vi "Loan_Calculator.vi"() -> ()   [LabVIEW 2022 SP3]
panel:
  in  "Loan Amount":dbl format="$ %#_g"
  in  "Compound Frequency":u16(ring) items=["Monthly", "Daily", "Continuously"]
  in  "Payment Frequency":dbl(ring) items=["Monthly"=12.0, "Quarterly"=4.0]
  out "Total Cost":dbl format="$ %#.2f"
  out "Payment Amount":dbl format="$ %#_g"
  in  "Years":dbl
  in  "Down Payment":dbl format="$ %#_g"
  in  "APR (%)":dbl
  # "Loan Calculator:\nInput a loan amount, the APR percentage, downpayment\namount, and length of the loan. Payment amount and total\nloan cost will be displayed on the right."
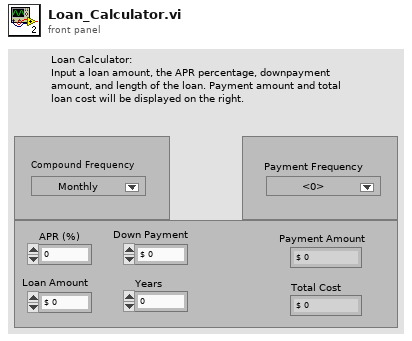
[diagram p1: front panel]
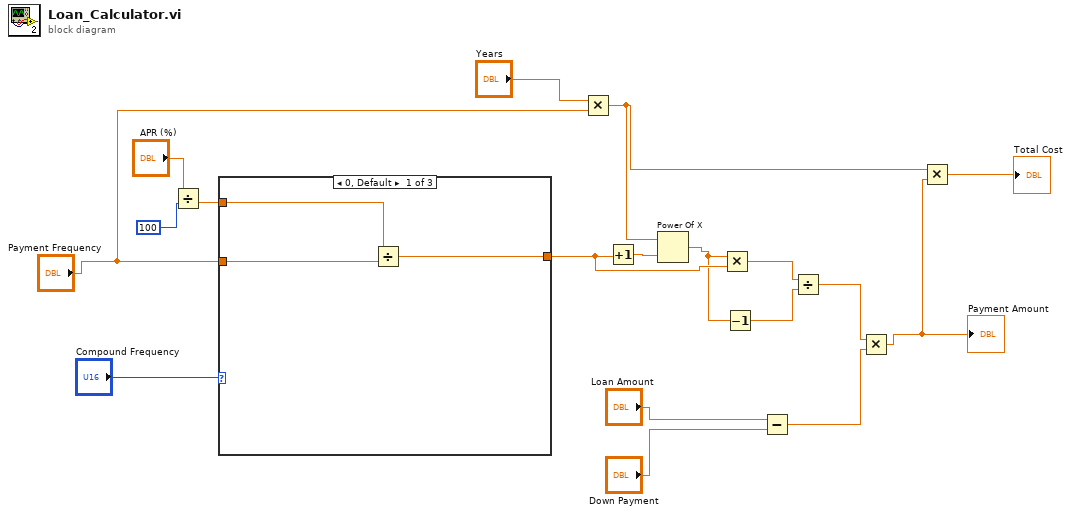
[diagram p0: block diagram]
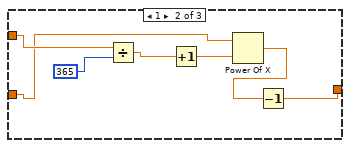
[diagram p2: hidden frame]
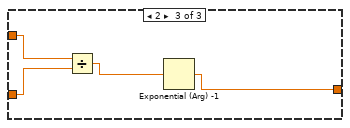
[diagram p3: hidden frame]
diagram:
  n1 = Divide(x="APR (%)", y=100) -> (x/y=w5:dbl)
  n2 = case shown="0, Default" "Compound Frequency" {
    tunnel: w5 -> [w21 w28 w32]
    tunnel: [w20 w23 w29] -> w17
    tunnel: "Payment Frequency" -> [w19 w25 w31]
    frame 0, Default {
      n3 = Divide(x=w21, y=w19) -> (x/y=w20:dbl)
    }
    frame 1 {
      n4 = Divide(x=w28, y=365) -> (x/y=w26:dbl)
      n5 = Increment(x=w26) -> (x+1=w24:dbl)
      n6 = Power Of X(1:w24, 2:w25) -> (0:w22:dbl)
      n7 = Decrement(x=w22) -> (x-1=w23:dbl)
    }
    frame 2 {
      n8 = Divide(x=w32, y=w31) -> (x/y=w30:dbl)
      n9 = Exponential (Arg) -1(1:w30) -> (0:w29:dbl)
    }
  }
  n10 = Multiply(x="Years", y="Payment Frequency") -> (x*y=w2:dbl)
  n11 = Increment(x=w17) -> (x+1=w18:dbl)
  n12 = Power Of X(1:w18, 2:w2) -> (0:w10:dbl)
  n13 = Multiply(x=w10, y=w17) -> (x*y=w12:dbl)
  n14 = Decrement(x=w10) -> (x-1=w11:dbl)
  n15 = Subtract(x="Loan Amount", y="Down Payment") -> (x-y=w7:dbl)
  n16 = Divide(x=w12, y=w11) -> (x/y=w6:dbl)
  n17 = Multiply(x=w6, y=w7) -> (x*y=w1:dbl)
  "Payment Amount" <- w1
  n18 = Multiply(x=w2, y=w1) -> (x*y=→"Total Cost":dbl)
